vi "VisualizeCHROMA0.vi"() -> ()   [LabVIEW 2018, in "Visualization.lvlib" / "VisualizeAcPwr.lvclass"]
uses:
  VisualizeAcPwr.lvclass
  VisualizeBase/VisualizeBase_class/Requests/clUserEventType.ctl
  <vilib>/event_ctls.llb/usereventprio.ctl
  <vilib>/Utility/error.llb/Error Cluster From Error Code.vi
  <vilib>/ErrorRing/Error Ring.xnode
  VisualizeBase/VisualizeBase_class/VisualizeBase.lvclass
  <userlib>/NIST/NISTErrorLib/NISTErrorLib.lvlib
  AcPwr/AcPwrModule/AcPwrModule.lvlib
panel:
  out "Chroma's Internal Errors/Warnings":string="No Error"
  out "Incorrect DataType?":bool
  in  "PluginName":string="AcPwr.Chroma0"
  in  "PlotYAxis":u32[](array[numeric])=[0, 1, 0] max=1
  out "Chroma":waveform(dbl)[](graph)=[{"t0"=timestamp(3657200531.6397257 s since 1904-01-01), "dt"=1.0, "Y"=[46.19]}, {"t0"=timestamp(3657200531.6397257 s since 1904-01-01), "dt"=1.0, "Y"=[2.0]}, {"t0"=timestamp(3657200531.6397257 s since 1904-01-01), "dt"=1.0, "Y"=[60.0]}]
  out "ErrorArray":errorcluster[](array[cluster])
  in  "QueuName":string="CHROMADCVQ"
  in  "btnStop":bool
  in  "btnReset":bool
  in  "btnClear":bool
  # "0=Left Axis and 1=Right Axis"
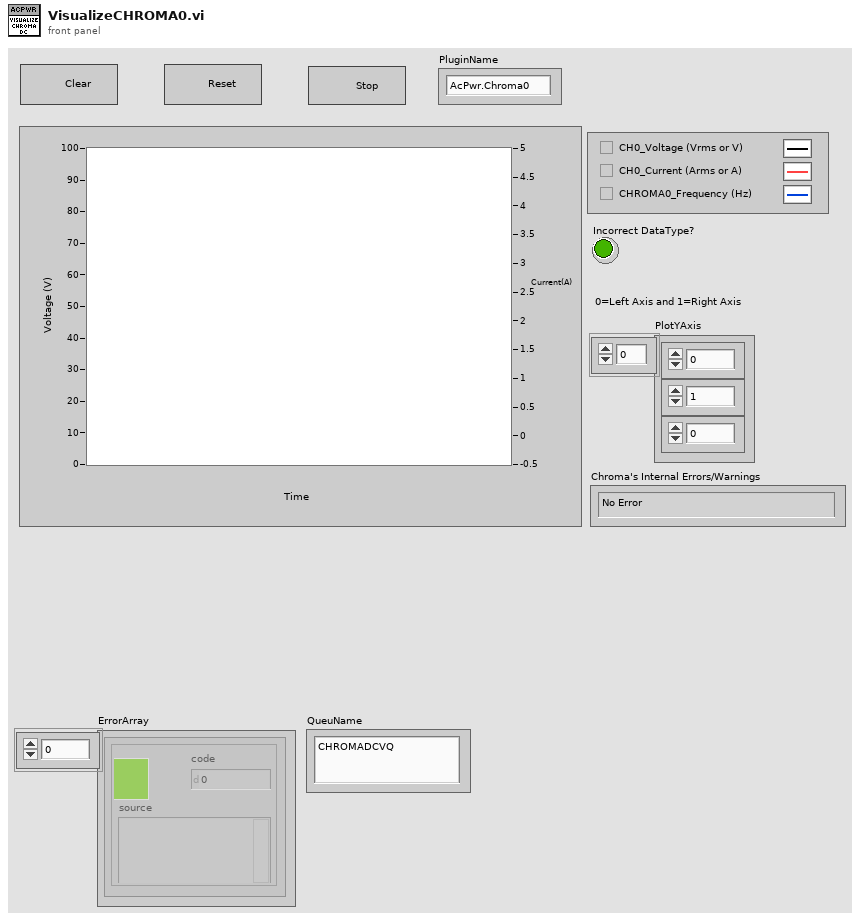
[diagram p1: front panel]
types:
  T1 = typedef "Visualization.lvlib/VisualizeBase.lvclass/clRequestEvents.ctl" = cluster{"StopRequest":refnum<user-event>, "ResetRequest":refnum<user-event>}
  T2 = typedef "AcPwrModule.lvlib/clBroadcastEvents.ctl" = cluster{"DidInit":refnum<user-event>, "StatusUpdate":refnum<user-event>, "ErrorReport":refnum<user-event>, "DidStop":refnum<user-event>, "PathToINI":refnum<user-event>, "Measurements":refnum<user-event>, "LoadConfigFile":refnum<user-event>, "GetSettings":refnum<user-event>, "SetSettings":refnum<user-event>, "GetType&ID":refnum<user-event>, "GotSettings":refnum<user-event>}
  T3 = typedef "Visualization.lvlib/VisualizeBase.lvclass/clUserEventType.ctl" = cluster{"BusIndex":i8, "Data":variant}
  T4 = typedef "usereventprio.ctl" = enum32{"high priority", "normal priority"}
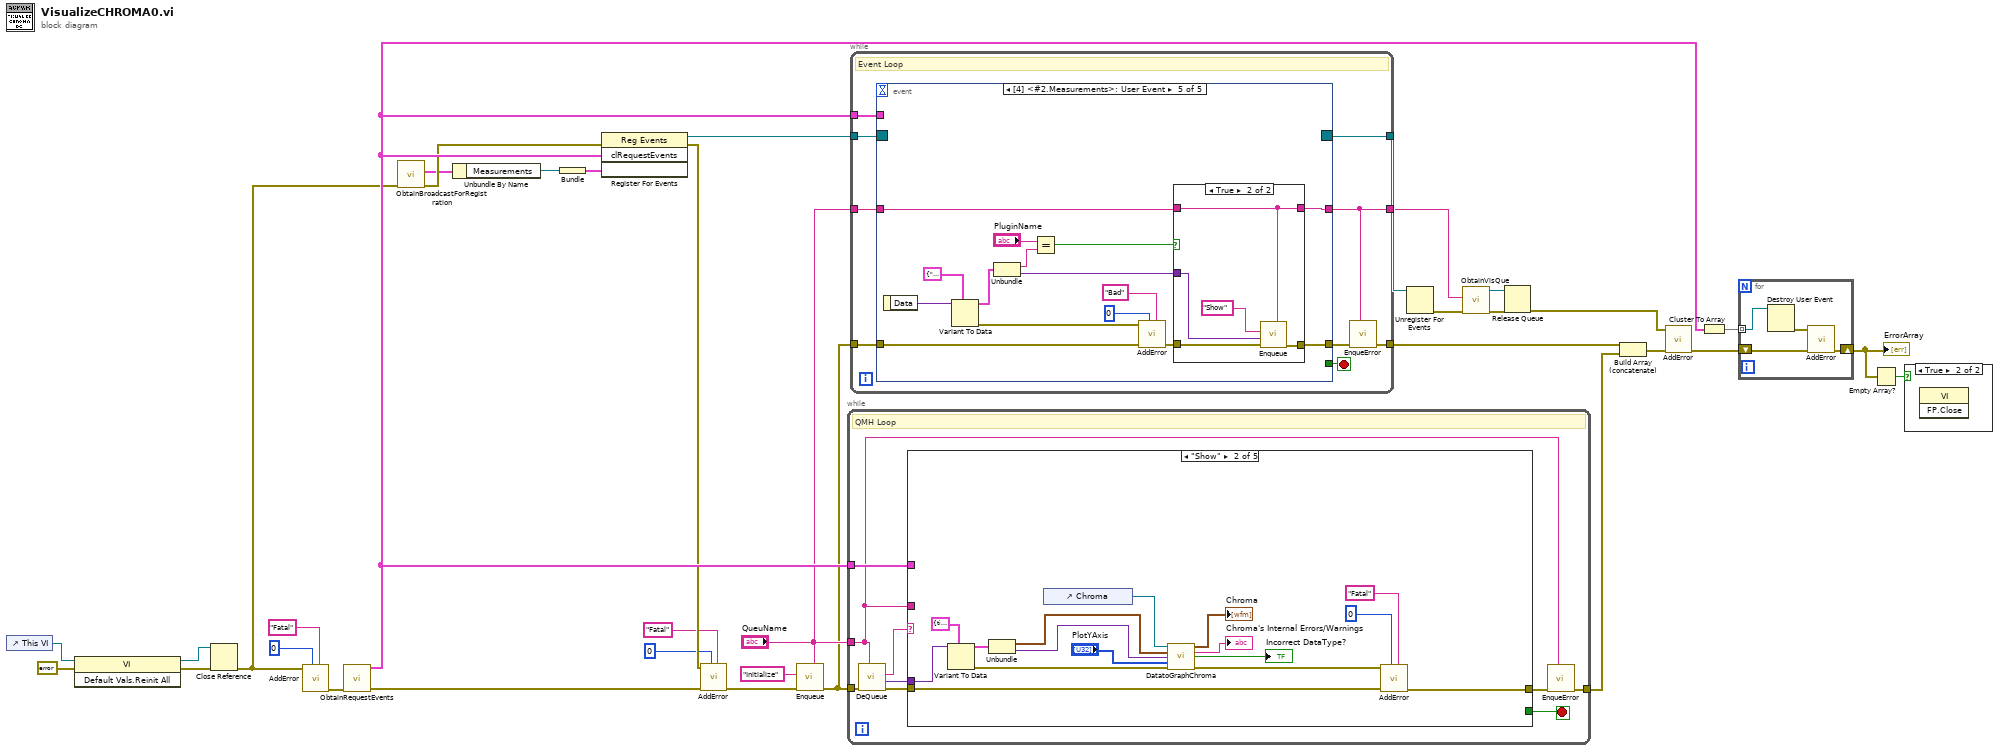
[diagram p0: block diagram]
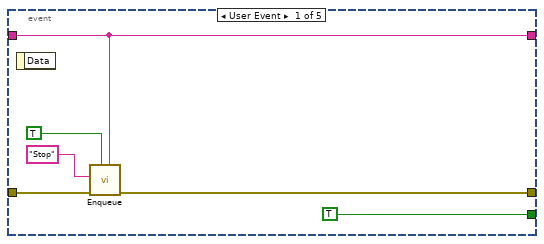
[diagram p2: hidden frame]
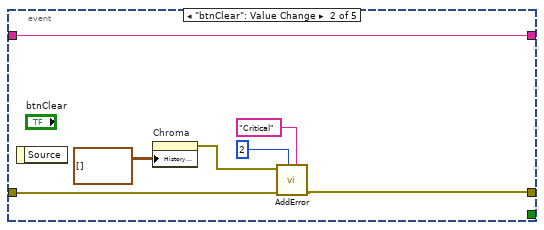
[diagram p3: hidden frame]
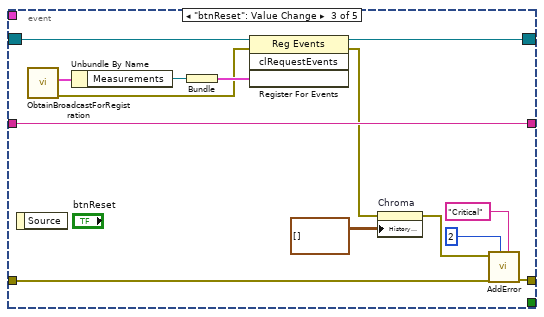
[diagram p4: hidden frame]
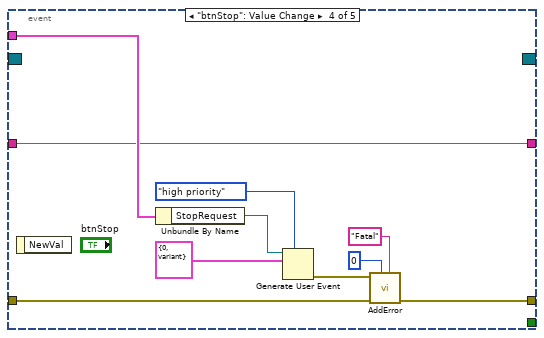
[diagram p5: hidden frame]
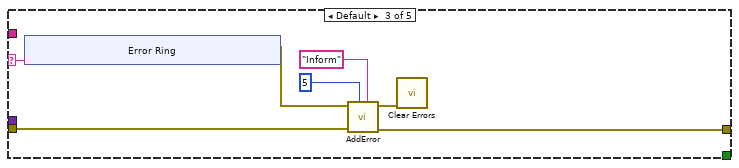
[diagram p8: hidden frame]
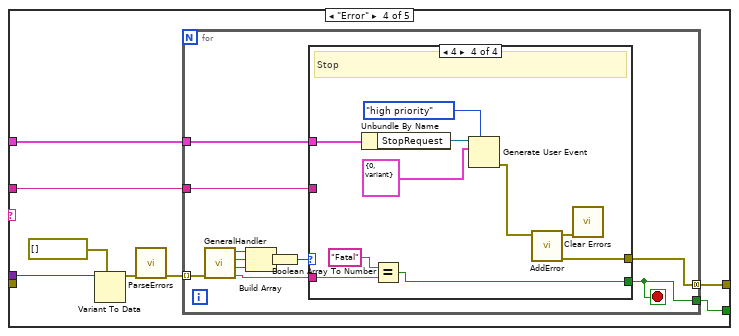
[diagram p9: hidden frame]
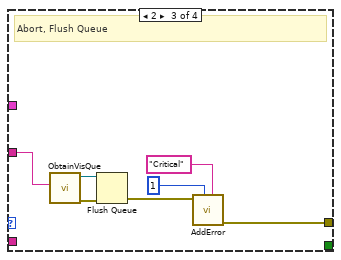
[diagram p12: hidden frame]
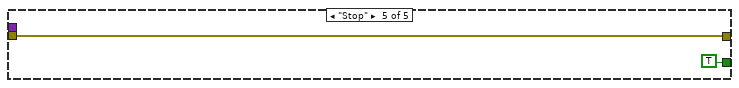
[diagram p13: hidden frame]
diagram:
  n1 = control-ref of="This VI"() -> (w18:refnum<vi>)
  n2 = invoke class="VI" method="Default Vals.Reinit All"(reference=w18, error in=errorcluster {"status"=FALSE, "code"=0, "source"=""} ("error in (no error)")) -> (reference out=w15:refnum<vi>, error out=w16:errorcluster)  [unwired: 1 in, 1 out]
  n3 = Close Reference(reference=w15, error in (no error)=w16) -> (error out=w13:errorcluster)
  n4 = call <userlib>:"AddError.vi"("Severity"="Fatal", "Priority"=u8 0, "error in (no error)"=w13) -> ("ErrorArray"=w33:errorcluster[])  [unwired: 7 in, 1 out]
  n5 = call "ObtainRequestEvents.vi"("Error"=w33) -> ("Error"=w7:errorcluster[], "clRequestEvents"=w22:T1)  [unwired: 9 in]
  n6 = call "ObtainBroadcastForRegistration.vi"("error in (no error)"=w13) -> ("error out"=w12:errorcluster, "clBroadcastEvents"=w11:T2)  [unwired: 9 in]
  n7 = Unbundle By Name(w11) -> ("Measurements"=w20:refnum<user-event>)
  n8 = Bundle("Measurements"=w20) -> (w19:cluster{"Measurements":refnum<user-event>})  [unwired: 1 in]
  n9 = register-events(error in=w12, w22, w19) -> (reference out=w34:refnum<event-registration>, error out=w4:errorcluster)  [unwired: 1 in]
  n10 = call <userlib>:"AddError.vi"("Severity"="Fatal", "Priority"=u8 0, "ErrorArray"=w7, "error in (no error)"=w4) -> ("ErrorArray"=w6:errorcluster[])  [unwired: 6 in, 1 out]
  n11 = call "Enqueue.vi"("QueName"="QueuName", "Error"=w6, "Message"="Initialize") -> ("Error"=w1:errorcluster[])  [unwired: 8 in]
  n12 = while {
    tunnel: w1 -> [w44]
    tunnel: [w38] -> w29
    tunnel: "QueuName" -> [w36]
    tunnel: w22 -> [w37]
    stop <- w39 stop-if-true
    # "QMH Loop"
    n13 = call "DeQueue.vi"("QueName"=w36, "Error"=w44) -> ("Error"=w41:errorcluster[], "Data"=w42:variant, "Message"=w43:string)  [unwired: 7 in]
    n14 = case shown="\"Show\"" w43 {
      selector: w43 -> [_ _ w68 _ _]
      tunnel: w42 -> [_ w57 _ w83 _]
      tunnel: w41 -> [w45 w54 w66 _ w112]
      tunnel: [w45 w61 w65 w79 w112] -> w40
      tunnel: [_ _ _ w78 TRUE] -> w39
      tunnel: w37 -> [_ _ _ w77 _]
      tunnel: w36 -> [_ _ _ w76 _]
      frame "Initialize" {
      }
      frame "Show" {
        n15 = Variant To Data(type=cluster{timestamp, "Data":variant} {timestamp(0 s since 1904-01-01), "Data"=variant}, Variant=w57) -> (data=w58:cluster{timestamp, "Data":variant}, error out=w56:errorcluster)  [unwired: 1 in]
        n16 = Unbundle(w58) -> (w47:timestamp, "Data"=w46:variant)
        n17 = control-ref of="Chroma"() -> (w59:refnum<vi>)
        n18 = call "DatatoGraphChroma.vi"("WaveformChartReference"=w59, "Time Stamp"=w47, "Data"=w46, "PlotYScale"="PlotYAxis", "error in (no error)"=w56) -> ("WaveformArray"=→"Chroma":waveform(dbl)[], "OutputString"=→"Chroma's Internal Errors/Warnings":string, "Incorrect DataType?"=→"Incorrect DataType?":bool, "error out"=w53:errorcluster)  [unwired: 7 in]
        n19 = call <userlib>:"AddError.vi"("Severity"="Fatal" ("String"), "Priority"=u8 0, "ErrorArray"=w54, "error in (no error)"=w53) -> ("ErrorArray"=w61:errorcluster[])  [unwired: 6 in, 1 out]
      }
      frame Default {
        n20 = xnode "Error Ring"("parameter 0"=w68) -> ("error out"=w67:errorcluster)
        n21 = call <userlib>:"AddError.vi"("Severity"="Inform" ("String"), "Priority"=u8 5, "ErrorArray"=w66, "error in (no error)"=w67) -> ("ErrorArray"=w65:errorcluster[], "error out"=w64:errorcluster)  [unwired: 6 in]
        n22 = call <vilib>:"Clear Errors.vi"("error in (no error)"=w64) -> ()  [unwired: 5 in, 2 out]
      }
      frame "Error" {
        n23 = Variant To Data(type=errorcluster[] [], Variant=w83) -> (data=w81:errorcluster[])  [unwired: 1 in, 1 out]
        n24 = call <userlib>:"ParseErrors.vi"("ErrorArray"=w81) -> ("ErrorArray"=w80:errorcluster[])  [unwired: 8 in, 2 out]
        n25 = for {
          tunnel: w80 -> [w94] mode=indexing
          tunnel: [w88] -> w79 mode=concatenating
          tunnel: [w86] -> w78
          tunnel: w77 -> [w85]
          tunnel: w76 -> [w84]
          stop <- w86 stop-if-true
          n26 = call <userlib>:"GeneralHandler.vi"("error in (no error)"=w94) -> ("Severity"=w87:string, "Stop"=w91:bool, "Abort"=w92:bool, "Continue"=w93:bool)  [unwired: 7 in]
          n27 = Build Array(w93, w92, w91) -> (w90:bool[])
          n28 = Boolean Array To Number(Boolean array=w90) -> (number=w89:u32)
          n29 = case shown="4" w89 {
            tunnel: [_ _ w99 w110] -> w88
            tunnel: w87 -> [_ _ _ w105]
            tunnel: [_ _ _ w103] -> w86
            tunnel: w85 -> [_ _ _ w102]
            tunnel: w84 -> [_ _ w95 _]
            frame 0, Default {
              # "No Dialog"
            }
            frame 1 {
              # "Continue"
            }
            frame 2 {
              # "Abort, Flush Queue"
              n30 = call "ObtainVisQue.vi"("QueName"=w95) -> ("error out"=w101:errorcluster, "queue out"=w100:refnum<queue>)  [unwired: 9 in]
              n31 = Flush Queue(queue=w100, error in (no error)=w101) -> (error out=w98:errorcluster)  [unwired: 2 out]
              n32 = call <userlib>:"AddError.vi"("Severity"="Critical" ("String"), "Priority"=u8 1, "error in (no error)"=w98) -> ("ErrorArray"=w99:errorcluster[])  [unwired: 7 in, 1 out]
            }
            frame 4 {
              # "Stop"
              n33 = Unbundle By Name(w102) -> ("StopRequest"=w111:refnum<user-event>)
              n34 = Equal?(x="Fatal", y=w105) -> (x = y?=w103:bool)
              n35 = Generate User Event(priority (normal)=usereventprio."high priority", user event=w111, event data cluster=T3 {"BusIndex"=0, "Data"=variant} ("event data")) -> (error out=w109:errorcluster)  [unwired: 1 in, 1 out]
              n36 = call <userlib>:"AddError.vi"("error in (no error)"=w109) -> ("ErrorArray"=w110:errorcluster[], "error out"=w106:errorcluster)  [unwired: 9 in]
              n37 = call <vilib>:"Clear Errors.vi"("error in (no error)"=w106) -> ()  [unwired: 5 in, 2 out]
            }
          }
        }
      }
      frame "Stop" {
      }
    }
    n38 = call "EnqueError.vi"("QueName"=w36, "Error"=w40) -> ("Error"=w38:errorcluster[])  [unwired: 9 in]
  }
  n39 = while {
    tunnel: w34 -> [w122]
    tunnel: [w119] -> w30
    tunnel: [w118] -> w32
    tunnel: w22 -> [w117]
    tunnel: w1 -> [w116]
    tunnel: "QueuName" -> [w115]
    tunnel: [w114] -> w9
    stop <- w121 stop-if-true
    # "Event Loop"
    n40 = event shown="[4] <#2.Measurements>: User Event" {
      selector: w122 -> [_ _ w149 _ _]
      dyn-events: [_ _ w148 _ _] -> w118
      timeout: _ -> [_ _ _ _ _]
      tunnel: [TRUE _ _ _ _] -> w121
      tunnel: [w127 w131 w141 w157 w174] -> w120
      tunnel: w117 -> [_ _ _ w152 _]
      tunnel: w116 -> [w124 w132 w142 w150 w162]
      tunnel: w115 -> [w123 w135 w143 w151 w173]
      tunnel: [w123 w135 w143 w151 w165] -> w114
      event User Event {
        n41 = event-data() -> ()  [unwired: 1 in, 1 out]
        n42 = call "Enqueue.vi"("QueName"=w123, "Priority? (F)"=TRUE, "Error"=w124, "Message"="Stop") -> ("Error"=w127:errorcluster[])  [unwired: 7 in]
      }
      event "btnClear": Value Change {
        n43 = event-data() -> ()  [unwired: 1 in, 1 out]
        n44 = property on="Chroma" class="WFChart (strict)"("History Data"=waveform(dbl)[][] []) -> (error out=w130:errorcluster)  [unwired: 2 in, 1 out]
        n45 = call <userlib>:"AddError.vi"("Severity"="Critical", "Priority"=u8 2, "ErrorArray"=w132, "error in (no error)"=w130) -> ("ErrorArray"=w131:errorcluster[])  [unwired: 6 in, 1 out]
      }
      event "btnReset": Value Change {
        n46 = event-data() -> ()  [unwired: 1 in, 1 out]
        n47 = call "ObtainBroadcastForRegistration.vi"() -> ("error out"=w144:errorcluster, "clBroadcastEvents"=w145:T2)  [unwired: 10 in]
        n48 = Unbundle By Name(w145) -> ("Measurements"=w147:refnum<user-event>)
        n49 = Bundle("Measurements"=w147) -> (w146:cluster{"Measurements":refnum<user-event>})  [unwired: 1 in]
        n50 = register-events(reference=w149, error in=w144, w146) -> (reference out=w148:refnum<event-registration>, error out=w137:errorcluster)  [unwired: 1 in]
        n51 = property on="Chroma" class="WFChart (strict)"(error in=w137, "History Data"=waveform(dbl)[][] []) -> (error out=w136:errorcluster)  [unwired: 1 in, 1 out]
        n52 = call <userlib>:"AddError.vi"("Severity"="Critical", "Priority"=u8 2, "ErrorArray"=w142, "error in (no error)"=w136) -> ("ErrorArray"=w141:errorcluster[])  [unwired: 6 in, 1 out]
      }
      event "btnStop": Value Change {
        n53 = event-data() -> ()  [unwired: 1 in, 1 out]
        n54 = Unbundle By Name(w152) -> ("StopRequest"=w158:refnum<user-event>)
        n55 = Generate User Event(priority (normal)=usereventprio."high priority", user event=w158, event data cluster=T3 {"BusIndex"=0, "Data"=variant} ("event data")) -> (error out=w159:errorcluster)  [unwired: 1 in, 1 out]
        n56 = call <userlib>:"AddError.vi"("Severity"="Fatal" ("String"), "Priority"=u8 0, "ErrorArray"=w150, "error in (no error)"=w159) -> ("ErrorArray"=w157:errorcluster[])  [unwired: 6 in, 1 out]
      }
      event User Event {
        n57 = event-data() -> ("Data"=w171:variant)  [unwired: 1 in]
        n58 = Variant To Data(type=cluster{string, "Data":variant} {"", "Data"=variant}, Variant=w171) -> (data=w169:cluster{string, "Data":variant}, error out=w160:errorcluster)  [unwired: 1 in]
        n59 = Unbundle(w169) -> (w167:string, "Data"=w166:variant)
        n60 = Equal?(x="PluginName", y=w167) -> (x = y?=w172:bool)
        n61 = call <userlib>:"AddError.vi"("Severity"="Bad" ("String"), "Priority"=u8 0, "ErrorArray"=w162, "error in (no error)"=w160) -> ("ErrorArray"=w161:errorcluster[])  [unwired: 6 in, 1 out]
        n62 = case shown="True" w172 {
          tunnel: [w176 w180] -> w174
          tunnel: w173 -> [w175 w177]
          tunnel: w161 -> [w176 w179]
          tunnel: w166 -> [_ w178]
          tunnel: [w175 w177] -> w165
          frame False {
          }
          frame True {
            n63 = call "Enqueue.vi"("QueName"=w177, "Error"=w179, "Data"=w178, "Message"="Show") -> ("Error"=w180:errorcluster[])  [unwired: 7 in]
          }
        }
      }
    }
    n64 = call "EnqueError.vi"("QueName"=w114, "Error"=w120) -> ("Error"=w119:errorcluster[])  [unwired: 9 in]
  }
  n65 = Unregister For Events(event registration refnum=w32) -> (error out=w28:errorcluster)  [unwired: 1 in]
  n66 = call "ObtainVisQue.vi"("error in (no error)"=w28, "QueName"=w9) -> ("error out"=w26:errorcluster, "queue out"=w25:refnum<queue>)  [unwired: 8 in]
  n67 = Release Queue(queue=w25, error in (no error)=w26) -> (error out=w24:errorcluster)  [unwired: 1 in, 2 out]
  n68 = Build Array (concatenate)(w30, w29) -> (w27:errorcluster[])
  n69 = call <userlib>:"AddError.vi"("ErrorArray"=w27, "error in (no error)"=w24) -> ("ErrorArray"=w23:errorcluster[])  [unwired: 8 in, 1 out]
  n70 = Cluster To Array(cluster=w22) -> (array=w31:refnum<user-event>[])
  n71 = for {
    tunnel: w31 -> [w185] mode=indexing
    shift-right: [w184] -> w14
    shift-left: w23 -> [w183]
    n72 = Destroy User Event(user event=w185) -> (error out=w182:errorcluster)  [unwired: 1 in]
    n73 = call <userlib>:"AddError.vi"("ErrorArray"=w183, "error in (no error)"=w182) -> ("ErrorArray"=w184:errorcluster[])  [unwired: 8 in, 1 out]
  }
  "ErrorArray" <- w14
  n74 = Empty Array?(array=w14) -> (empty?=w21:bool)
  n75 = case shown="True" w21 {
    frame False {
    }
    frame True {
      n76 = invoke class="VI" method="FP.Close"() -> ()  [unwired: 3 in, 3 out]
    }
  }
